vi "CNR DogLeg step.vi"(5 "gradient":dbl[](array[numeric]) format="%.2f", 6 "Hessian":T1, 7 "TR radius":dbl format="%#_6e", 8 "error in (no error)":errorcluster) -> (0 "error out":errorcluster, 2 "L(0)-L(hdl)\npredicted change":dbl format="%#_10e", 3 "x step":dbl[](array[numeric]))   [LabVIEW 2010, in "NI_Gmath.lvlib"]
uses:
  NI_Gmath.lvlib
  RealMatrix.ctl
  Real Dot Product.vi
  A x Vector.vi
  NI_AALBase.lvlib
  NI_Matrix.lvlib
panel:
  in  "previous step accepted?":bool
  out "x = 0?":bool
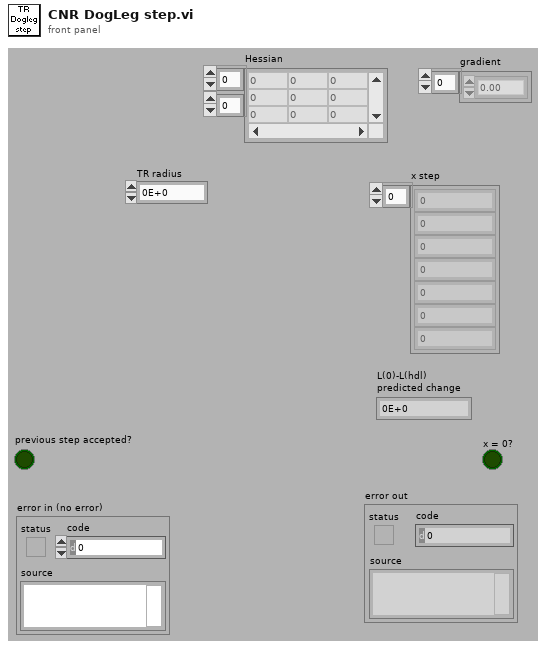
[diagram p1: front panel]
types:
  T1 = typedef "NI_Matrix.lvlib/RealMatrix.ctl" = dbl[][]
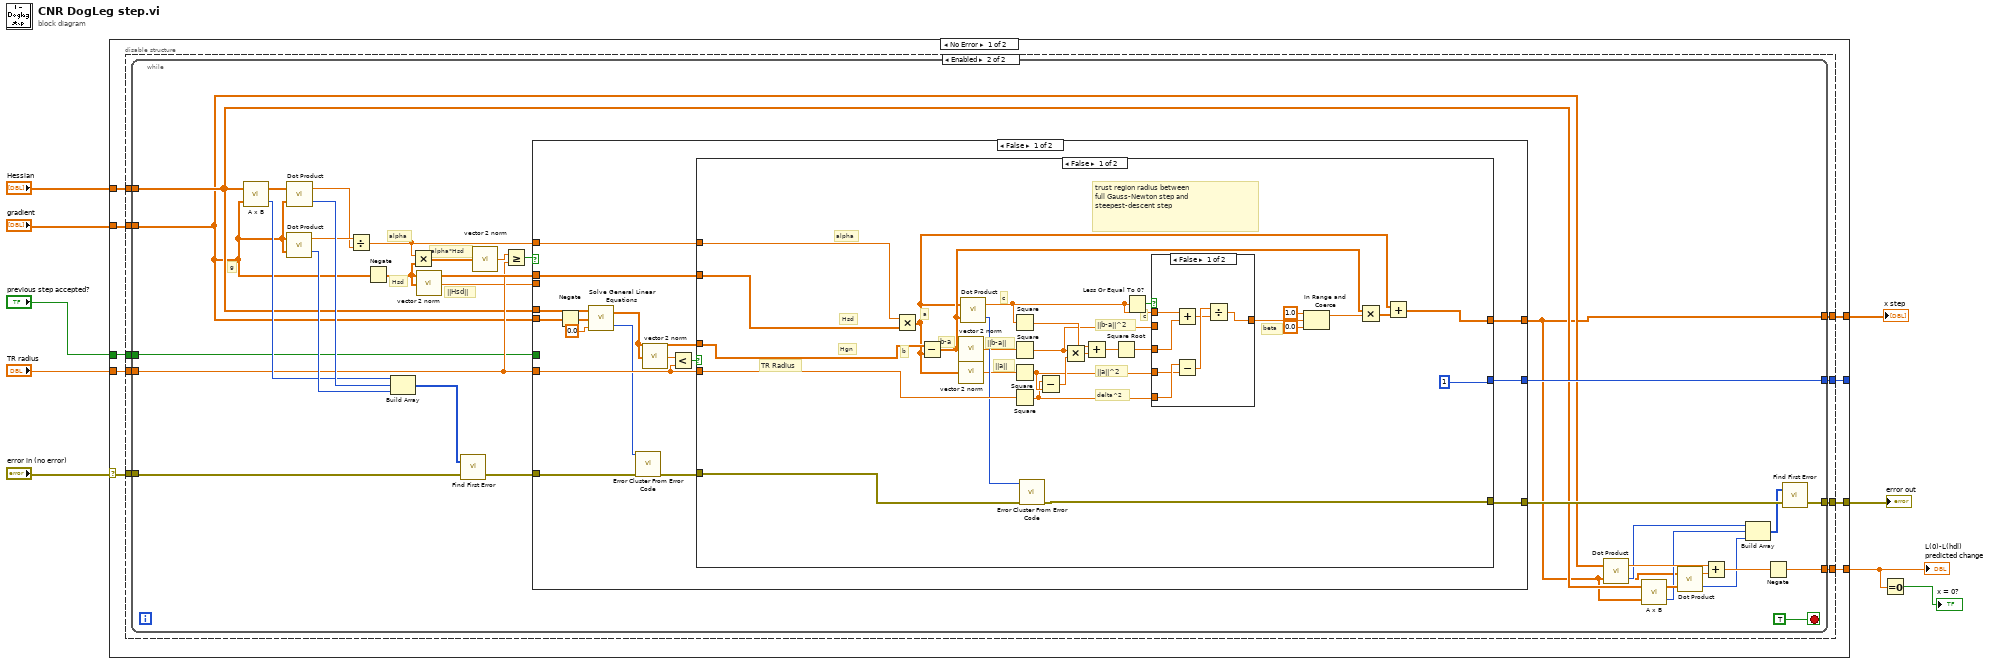
[diagram p0: block diagram]
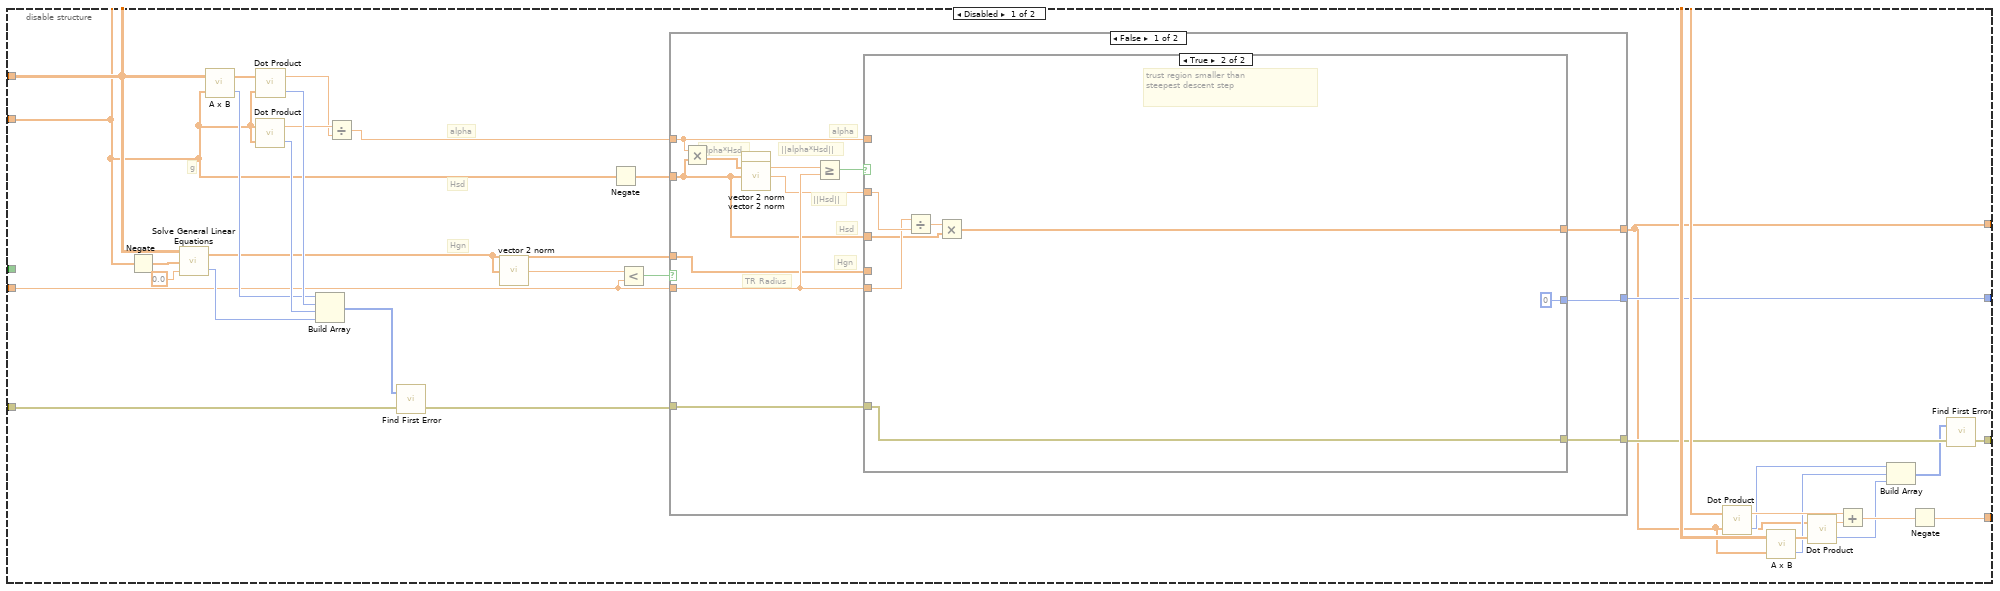
[diagram p2: hidden frame]
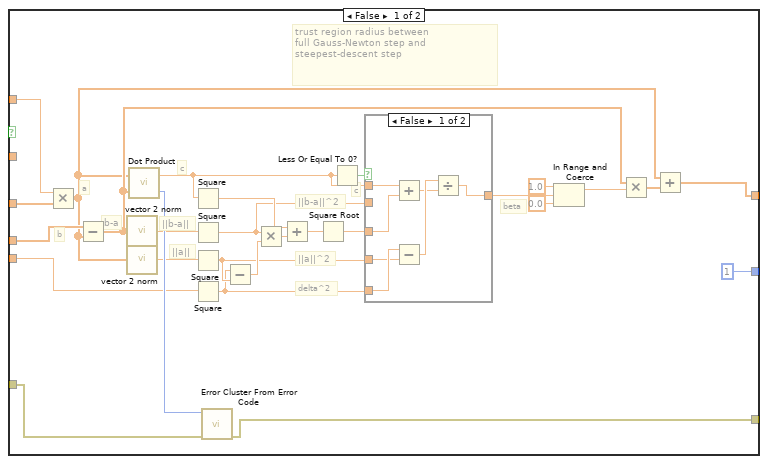
[diagram p3: hidden frame]
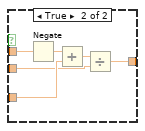
[diagram p4: hidden frame]
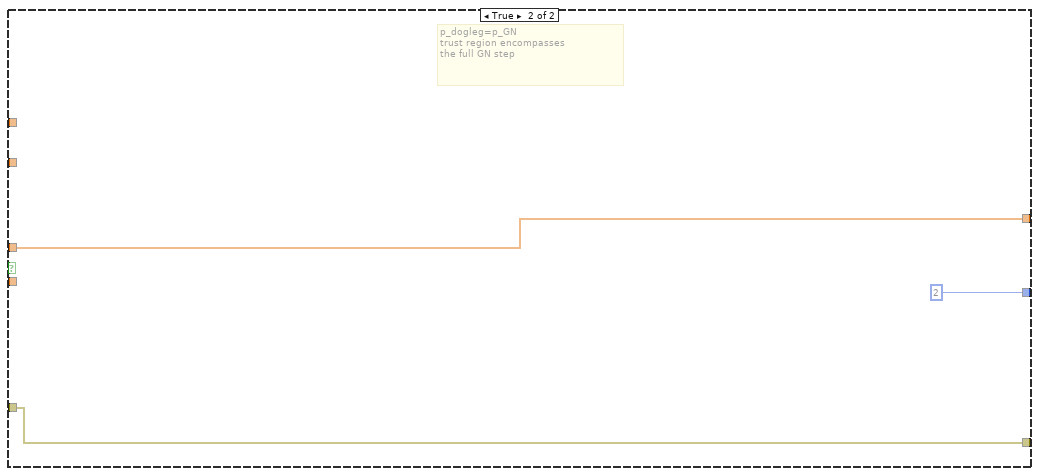
[diagram p5: hidden frame]
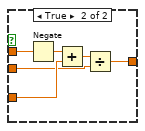
[diagram p6: hidden frame]
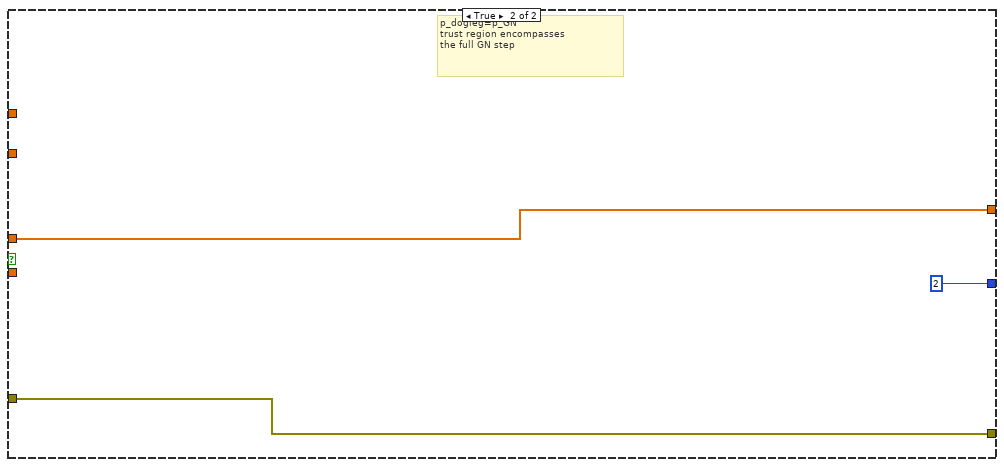
[diagram p7: hidden frame]
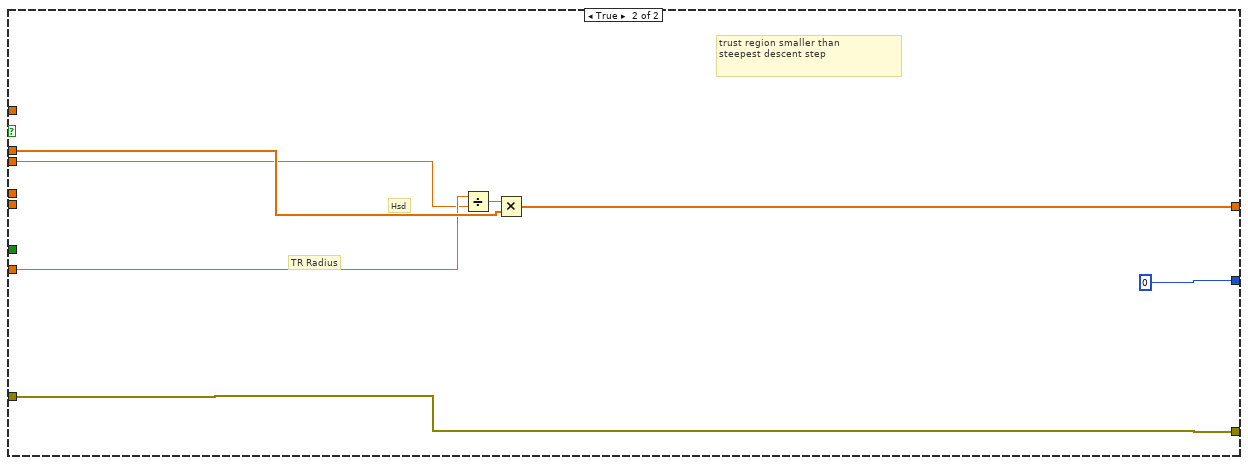
[diagram p8: hidden frame]
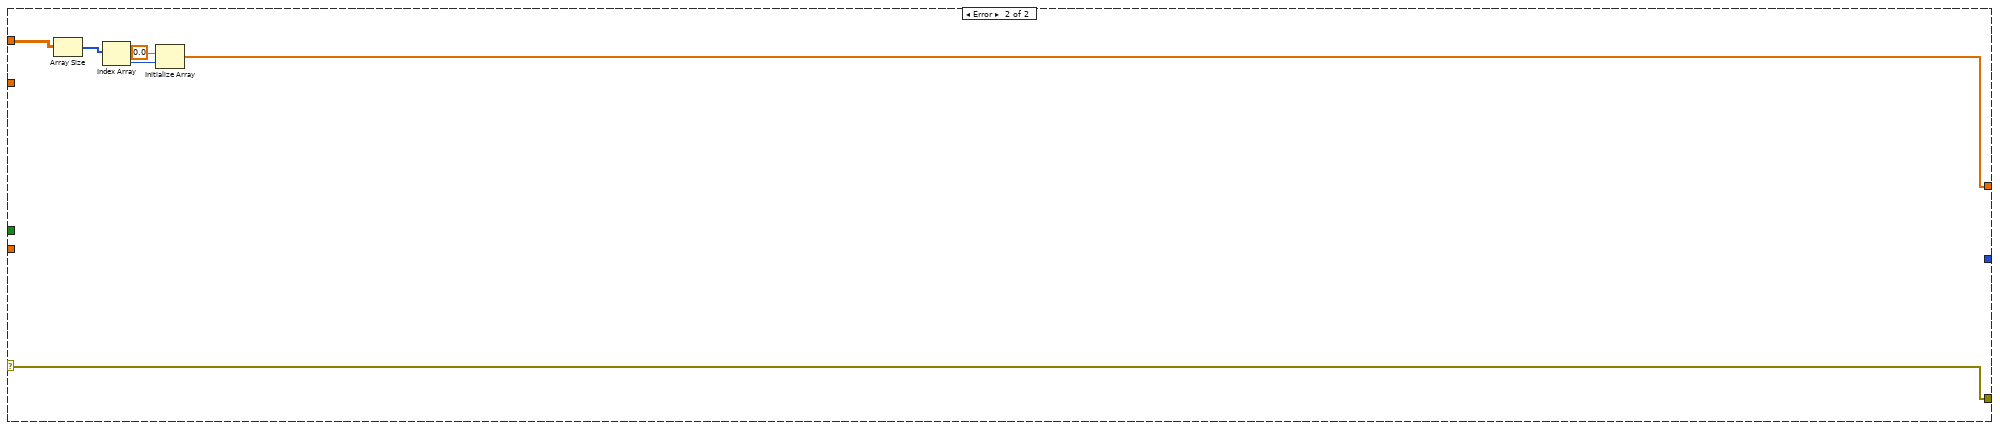
[diagram p9: hidden frame]
diagram:
  n1 = case shown="No Error" "error in (no error)" {
    selector: "error in (no error)" -> [w18 w229]
    tunnel: "TR radius" -> [w12 _]
    tunnel: [w13 w224] -> w8
    tunnel: [w15 w229] -> w6
    tunnel: [w14 _] -> _
    tunnel: "gradient" -> [w16 _]
    tunnel: "Hessian" -> [w17 w228]
    tunnel: [w11 _] -> w3
    tunnel: "previous step accepted?" -> [w10 _]
    frame No Error {
      n2 = disable-structure shown="Enabled" {
        disable-tunnel: w18 -> [w48 w123]
        disable-tunnel: w17 -> [w35 w122]
        disable-tunnel: w16 -> [w34 w121]
        disable-tunnel: [w29 w120] -> w15
        disable-tunnel: [w23 w119] -> w14
        disable-tunnel: [w19 w118] -> w13
        disable-tunnel: w12 -> [w22 w117]
        disable-tunnel: [w20 w116] -> w11
        disable-tunnel: w10 -> [_ w115]
        frame Disabled {
          # "Hgn"
          # "Hsd"
          # "alpha"
          # "g"
          n3 = Negate(x=w34) -> (-x=w40:dbl[])
          n4 = call "Solve General Linear Equations.vi"("relative tolerance"=0.0, "Known Vector"=w40, "Input Matrix"=w35) -> ("error"=w44:i32, "Solution Vector"=w43:dbl[])
          n5 = call-poly "A x B.vi"("Vector"=w34, "A"=w35) -> ("error"=w49:i32, "A x Vector"=w32:dbl[])
          n6 = call-poly "Dot Product.vi"("Y Vector"=w34, "X Vector"=w34) -> ("error"=w50:i32, "X * Y"=w31:dbl)
          n7 = call-poly "Dot Product.vi"("Y Vector"=w34, "X Vector"=w32) -> ("error"=w51:i32, "X * Y"=w30:dbl)
          n8 = Build Array(w49, w51, w50, w44) -> (w46:i32[])
          n9 = Divide(x=w31, y=w30) -> (x/y=w47:dbl)
          n10 = call "Find First Error.vi"("error in (no error)"=w48, "error codes"=w46) -> ("error out"=w45:errorcluster)  [unwired: 2 in, 1 out]
          n11 = call "vector 2 norm.vi"("vector"=w43) -> ("vector2_norm"=w41:dbl)  [unwired: 14 in]
          n12 = Negate(x=w34) -> (-x=w33:dbl[])
          n13 = Less?(x=w41, y=w22) -> (x < y?=w42:bool)
          n14 = case shown="False" w42 {
            tunnel: w43 -> [w61 w114]
            tunnel: w33 -> [w58 _]
            tunnel: [w62 w114] -> w19
            tunnel: w22 -> [w63 _]
            tunnel: w47 -> [w57 _]
            tunnel: w45 -> [w60 w113]
            tunnel: [w59 w113] -> w28
            tunnel: [w56 2] -> w23
            frame False {
              # "TR Radius"
              # "||alpha*Hsd||"
              # "Hsd"
              # "Hgn"
              # "alpha"
              # "alpha*Hsd"
              # "||Hsd||"
              n15 = Multiply(x=w57, y=w58) -> (x*y=w54:dbl[])
              n16 = call "vector 2 norm.vi"("vector"=w54) -> ("vector2_norm"=w53:dbl)  [unwired: 14 in]
              n17 = call "vector 2 norm.vi"("vector"=w58) -> ("vector2_norm"=w55:dbl)  [unwired: 14 in]
              n18 = Greater Or Equal?(x=w53, y=w63) -> (x >= y?=w52:bool)
              n19 = case shown="True" w52 {
                tunnel: w55 -> [_ w110]
                tunnel: w63 -> [w87 w109]
                tunnel: w58 -> [w90 w107]
                tunnel: [w71 w105] -> w62
                tunnel: w57 -> [w76 _]
                tunnel: w61 -> [w89 _]
                tunnel: w60 -> [w75 w111]
                tunnel: [w74 w111] -> w59
                tunnel: [1 0] -> w56
                frame False {
                  # "trust region radius between\nfull Gauss-Newton step and \nsteepest-descent step"
                  # "beta"
                  # "delta^2"
                  # "c"
                  # "||b-a||^2"
                  # "||a||^2"
                  # "||b-a||"
                  # "||a||"
                  # "c"
                  # "b-a"
                  # "a"
                  # "b"
                  n20 = Multiply(x=w76, y=w90) -> (x*y=w72:dbl[])
                  n21 = Subtract(x=w89, y=w72) -> (x-y=w73:dbl[])
                  n22 = call "vector 2 norm.vi"("vector"=w73) -> ("vector2_norm"=w69:dbl)  [unwired: 14 in]
                  n23 = call "vector 2 norm.vi"("vector"=w72) -> ("vector2_norm"=w68:dbl)  [unwired: 14 in]
                  n24 = call-poly "Dot Product.vi"("Y Vector"=w73, "X Vector"=w72) -> ("error"=w91:i32, "X * Y"=w77:dbl)
                  n25 = Square(x=w77) -> (x^2=w84:dbl)
                  n26 = Square(x=w69) -> (x^2=w80:dbl)
                  n27 = Square(x=w68) -> (x^2=w81:dbl)
                  n28 = Square(x=w87) -> (x^2=w79:dbl)
                  n29 = call "Error Cluster From Error Code.vi"("error in (no error)"=w75, "error code (0)"=w91) -> ("error out"=w74:errorcluster)  [unwired: 7 in]
                  n30 = Subtract(x=w79, y=w81) -> (x-y=w86:dbl)
                  n31 = Multiply(x=w80, y=w86) -> (x*y=w85:dbl)
                  n32 = Add(x=w84, y=w85) -> (x+y=w83:dbl)
                  n33 = Square Root(x=w83) -> (sqrt(x)=w82:dbl)
                  n34 = Less Or Equal To 0?(x=w77) -> (x <= 0?=w88:bool)
                  n35 = case shown="False" w88 {
                    tunnel: w82 -> [w95 w102]
                    tunnel: w81 -> [w97 _]
                    tunnel: w80 -> [_ w100]
                    tunnel: w77 -> [w96 w104]
                    tunnel: [w92 w99] -> w64
                    tunnel: w79 -> [w98 _]
                    frame False {
                      n36 = Add(x=w96, y=w95) -> (x+y=w93:dbl)
                      n37 = Subtract(x=w98, y=w97) -> (x-y=w94:dbl)
                      n38 = Divide(x=w94, y=w93) -> (x/y=w92:dbl)
                    }
                    frame True {
                      n39 = Negate(x=w104) -> (-x=w103:dbl)
                      n40 = Add(x=w103, y=w102) -> (x+y=w101:dbl)
                      n41 = Divide(x=w101, y=w100) -> (x/y=w99:dbl)
                    }
                  }
                  n42 = In Range and Coerce(upper limit=1.0, x=w64, lower limit=0.0) -> (coerced(x)=w65:dbl)  [unwired: 1 out]
                  n43 = Multiply(x=w73, y=w65) -> (x*y=w78:dbl[])
                  n44 = Add(x=w72, y=w78) -> (x+y=w71:dbl[])
                }
                frame True {
                  # "trust region smaller than \nsteepest descent step"
                  n45 = Divide(x=w109, y=w110) -> (x/y=w108:dbl)
                  n46 = Multiply(x=w108, y=w107) -> (x*y=w105:dbl[])
                }
              }
            }
            frame True {
              # "p_dogleg=p_GN\ntrust region encompasses\nthe full GN step"
            }
          }
          n47 = call-poly "Dot Product.vi"("Y Vector"=w19, "X Vector"=w34) -> ("error"=w25:i32, "X * Y"=w37:dbl)
          n48 = call-poly "A x B.vi"("Vector"=w19, "A"=w35) -> ("error"=w26:i32, "A x Vector"=w39:dbl[])
          n49 = call-poly "Dot Product.vi"("Y Vector"=w39, "X Vector"=w19) -> ("error"=w27:i32, "X * Y"=w38:dbl)
          n50 = Add(x=w37, y=w38) -> (x+y=w36:dbl)
          n51 = Build Array(w25, w26, w27) -> (w24:i32[])
          n52 = Negate(x=w36) -> (-x=w20:dbl)
          n53 = call "Find First Error.vi"("error in (no error)"=w28, "error codes"=w24) -> ("error out"=w29:errorcluster)  [unwired: 2 in, 1 out]
        }
        frame Enabled {
          n54 = while {
            tunnel: w123 -> [w153]
            tunnel: w122 -> [w127]
            tunnel: w121 -> [w126]
            tunnel: [w143] -> w120
            tunnel: [w137] -> w119
            tunnel: [w124] -> w118
            tunnel: w117 -> [w131]
            tunnel: [w136] -> w116
            tunnel: w115 -> [w125]
            stop <- TRUE stop-if-true
            # "||Hsd||"
            # "alpha*Hsd"
            # "Hsd"
            # "alpha"
            # "g"
            n55 = call-poly "A x B.vi"("Vector"=w126, "A"=w127) -> ("error"=w154:i32, "A x Vector"=w146:dbl[])
            n56 = call-poly "Dot Product.vi"("Y Vector"=w126, "X Vector"=w126) -> ("error"=w155:i32, "X * Y"=w145:dbl)
            n57 = call-poly "Dot Product.vi"("Y Vector"=w126, "X Vector"=w146) -> ("error"=w156:i32, "X * Y"=w144:dbl)
            n58 = Divide(x=w145, y=w144) -> (x/y=w135:dbl)
            n59 = Negate(x=w126) -> (-x=w133:dbl[])
            n60 = Build Array(w154, w156, w155) -> (w152:i32[])
            n61 = Multiply(x=w135, y=w133) -> (x*y=w134:dbl[])
            n62 = call "vector 2 norm.vi"("vector"=w133) -> ("vector2_norm"=w129:dbl)  [unwired: 14 in]
            n63 = call "Find First Error.vi"("error in (no error)"=w153, "error codes"=w152) -> ("error out"=w151:errorcluster)  [unwired: 2 in, 1 out]
            n64 = call "vector 2 norm.vi"("vector"=w134) -> ("vector2_norm"=w132:dbl)  [unwired: 14 in]
            n65 = Greater Or Equal?(x=w132, y=w131) -> (x >= y?=w130:bool)
            n66 = case shown="False" w130 {
              tunnel: w151 -> [w161 w222]
              tunnel: [w172 w223] -> w124
              tunnel: [w171 w222] -> w142
              tunnel: [w170 0] -> w137
              tunnel: w135 -> [w169 _]
              tunnel: w133 -> [w168 w220]
              tunnel: w131 -> [w164 w219]
              tunnel: w129 -> [_ w217]
              tunnel: w127 -> [w167 _]
              tunnel: w126 -> [w166 _]
              tunnel: w125 -> [_ _]
              frame False {
                n67 = Negate(x=w166) -> (-x=w157:dbl[])
                n68 = call "Solve General Linear Equations.vi"("relative tolerance"=0.0, "Known Vector"=w157, "Input Matrix"=w167) -> ("error"=w159:i32, "Solution Vector"=w162:dbl[])
                n69 = call "Error Cluster From Error Code.vi"("error in (no error)"=w161, "error code (0)"=w159) -> ("error out"=w160:errorcluster)  [unwired: 7 in]
                n70 = call "vector 2 norm.vi"("vector"=w162) -> ("vector2_norm"=w165:dbl)  [unwired: 14 in]
                n71 = Less?(x=w165, y=w164) -> (x < y?=w163:bool)
                n72 = case shown="False" w163 {
                  tunnel: w162 -> [w198 w216]
                  tunnel: w168 -> [w195 _]
                  tunnel: [w199 w216] -> w172
                  tunnel: w164 -> [w200 _]
                  tunnel: w169 -> [w194 _]
                  tunnel: w160 -> [w197 w215]
                  tunnel: [w196 w215] -> w171
                  tunnel: [1 2] -> w170
                  frame False {
                    # "trust region radius between\nfull Gauss-Newton step and \nsteepest-descent step"
                    # "beta"
                    # "delta^2"
                    # "c"
                    # "||b-a||^2"
                    # "||a||^2"
                    # "||b-a||"
                    # "||a||"
                    # "c"
                    # "b-a"
                    # "a"
                    # "b"
                    # "TR Radius"
                    # "Hsd"
                    # "Hgn"
                    # "alpha"
                    n73 = Multiply(x=w194, y=w195) -> (x*y=w179:dbl[])
                    n74 = Subtract(x=w198, y=w179) -> (x-y=w180:dbl[])
                    n75 = call "vector 2 norm.vi"("vector"=w180) -> ("vector2_norm"=w178:dbl)  [unwired: 14 in]
                    n76 = call "vector 2 norm.vi"("vector"=w179) -> ("vector2_norm"=w177:dbl)  [unwired: 14 in]
                    n77 = call-poly "Dot Product.vi"("Y Vector"=w180, "X Vector"=w179) -> ("error"=w192:i32, "X * Y"=w181:dbl)
                    n78 = Square(x=w181) -> (x^2=w188:dbl)
                    n79 = Square(x=w178) -> (x^2=w184:dbl)
                    n80 = Square(x=w177) -> (x^2=w185:dbl)
                    n81 = Square(x=w200) -> (x^2=w183:dbl)
                    n82 = call "Error Cluster From Error Code.vi"("error in (no error)"=w197, "error code (0)"=w192) -> ("error out"=w196:errorcluster)  [unwired: 7 in]
                    n83 = Subtract(x=w183, y=w185) -> (x-y=w190:dbl)
                    n84 = Multiply(x=w184, y=w190) -> (x*y=w189:dbl)
                    n85 = Add(x=w188, y=w189) -> (x+y=w187:dbl)
                    n86 = Square Root(x=w187) -> (sqrt(x)=w186:dbl)
                    n87 = Less Or Equal To 0?(x=w181) -> (x <= 0?=w191:bool)
                    n88 = case shown="False" w191 {
                      tunnel: w186 -> [w204 w211]
                      tunnel: w185 -> [w206 _]
                      tunnel: w184 -> [_ w209]
                      tunnel: w181 -> [w205 w213]
                      tunnel: [w201 w208] -> w173
                      tunnel: w183 -> [w207 _]
                      frame False {
                        n89 = Add(x=w205, y=w204) -> (x+y=w202:dbl)
                        n90 = Subtract(x=w207, y=w206) -> (x-y=w203:dbl)
                        n91 = Divide(x=w203, y=w202) -> (x/y=w201:dbl)
                      }
                      frame True {
                        n92 = Negate(x=w213) -> (-x=w212:dbl)
                        n93 = Add(x=w212, y=w211) -> (x+y=w210:dbl)
                        n94 = Divide(x=w210, y=w209) -> (x/y=w208:dbl)
                      }
                    }
                    n95 = In Range and Coerce(upper limit=1.0, x=w173, lower limit=0.0) -> (coerced(x)=w174:dbl)  [unwired: 1 out]
                    n96 = Multiply(x=w180, y=w174) -> (x*y=w182:dbl[])
                    n97 = Add(x=w179, y=w182) -> (x+y=w199:dbl[])
                  }
                  frame True {
                    # "p_dogleg=p_GN\ntrust region encompasses\nthe full GN step"
                  }
                }
              }
              frame True {
                # "trust region smaller than \nsteepest descent step"
                # "TR Radius"
                # "Hsd"
                n98 = Divide(x=w219, y=w217) -> (x/y=w218:dbl)
                n99 = Multiply(x=w218, y=w220) -> (x*y=w223:dbl[])
              }
            }
            n100 = call-poly "Dot Product.vi"("Y Vector"=w124, "X Vector"=w126) -> ("error"=w139:i32, "X * Y"=w148:dbl)
            n101 = call-poly "A x B.vi"("Vector"=w124, "A"=w127) -> ("error"=w140:i32, "A x Vector"=w150:dbl[])
            n102 = call-poly "Dot Product.vi"("Y Vector"=w150, "X Vector"=w124) -> ("error"=w141:i32, "X * Y"=w149:dbl)
            n103 = Add(x=w148, y=w149) -> (x+y=w147:dbl)
            n104 = Build Array(w139, w140, w141) -> (w138:i32[])
            n105 = Negate(x=w147) -> (-x=w136:dbl)
            n106 = call "Find First Error.vi"("error in (no error)"=w142, "error codes"=w138) -> ("error out"=w143:errorcluster)  [unwired: 2 in, 1 out]
          }
        }
      }
    }
    frame Error {
      n107 = Array Size(array=w228) -> (size(s)=w227:i32[])
      n108 = Index Array(array=w227) -> (element=w226:i32)  [unwired: 1 in]
      n109 = Initialize Array(0.0 ("element"), w226) -> (w224:dbl[])
    }
  }
  "x step" <- w8
  "error out" <- w6
  "L(0)-L(hdl)\npredicted change" <- w3
  n110 = Equal To 0?(x=w3) -> (x = 0?=→"x = 0?":bool)
